vi "PH_Beckhoff_PP_PU.set GUI Elements to Default.vi"(0 "i ref in":refnum<vi>, 5 "error in":errorcluster) -> (14 "i ref out":refnum<vi>, 19 "error out":errorcluster)   [LabVIEW 2014, in "PH_Beckhoff_PP_PU.lvlib"]
doc: "Within this VI captions are set and GUI elements which are not in use are set not to be visible."
uses:
  PH_Beckhoff_PP_PU.lvlib
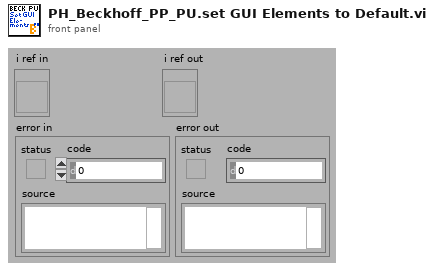
[diagram p1: front panel]
types:
  T1 = typedef "PH_Beckhoff_PP_PU.lvlib/PH_Beckhoff_PP_PU.PU Rack Type.ctl" = enum16{"no Info", "PA 19mm", "PA 45mm", "MA PU 1 and 2", "MA PU 3 and 4", "MA PU 5 and 6", "MA FR and PILC"}
  T2 = typedef "PH_PP_Common.lvlib/PH_PP_Common.PUs.ctl" = enum16{"no Info", "PA-19mm-1", "PA-19mm-2", "PA-45mm-PILC", "PA-45mm-MAIN", "MA-PU-1", "MA-PU-2", "MA-PU-3", "MA-PU-4", "MA-PU-5", "MA-PU-6", "MA-FR", "MA-PILC", "PA-45mm-DP"}
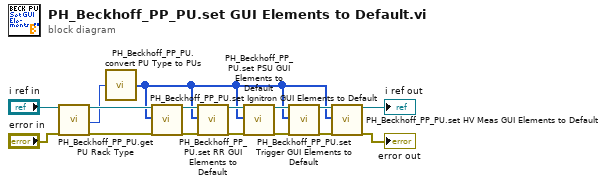
[diagram p0: block diagram]
diagram:
  n1 = call "PH_Beckhoff_PP_PU.get PU Rack Type.vi"("VI in"="i ref in", "error in (no error)"="error in") -> ("VI out"=w9:refnum<vi>, "PU Rack Type"=w1:T1, "error out"=w14:errorcluster)  [unwired: 15 in]
  n2 = call "PH_Beckhoff_PP_PU.convert PU Type to PUs.vi"("PU Type"=w1) -> ("PUs"=w2:T2[])
  n3 = call "PH_Beckhoff_PP_PU.set Ignitron GUI Elements to Default.vi"("i ref in"=w9, "PUs"=w2, "error in"=w14) -> ("i ref out"=w7:refnum<vi>, "error out"=w10:errorcluster)  [unwired: 15 in]
  n4 = call "PH_Beckhoff_PP_PU.set RR GUI Elements to Default.vi"("i ref in"=w7, "PUs"=w2, "error in"=w10) -> ("i ref out"=w6:refnum<vi>, "error out"=w8:errorcluster)  [unwired: 15 in]
  n5 = call "PH_Beckhoff_PP_PU.set PSU GUI Elements to Default.vi"("i ref in"=w6, "PUs"=w2, "error in"=w8) -> ("i ref out"=w4:refnum<vi>, "error out"=w12:errorcluster)  [unwired: 15 in]
  n6 = call "PH_Beckhoff_PP_PU.set Trigger GUI Elements to Default.vi"("i ref in"=w4, "PUs"=w2, "error in"=w12) -> ("i ref out"=w3:refnum<vi>, "error out"=w5:errorcluster)  [unwired: 15 in]
  n7 = call "PH_Beckhoff_PP_PU.set HV Meas GUI Elements to Default.vi"("i ref in"=w3, "PUs"=w2, "error in"=w5) -> ("i ref out"=→"i ref out":refnum<vi>, "error out"=→"error out":errorcluster)  [unwired: 15 in]
